vi "Queued Temperature Controller.vi"() -> ()   [LabVIEW 2013]
uses:
  Heater State.ctl
  <vilib>/Analysis/baseanly.llb/Mean (DBL).vi
  <vilib>/Analysis/NI_AALBase.lvlib
panel:
  out "Current Temperature":dbl
  out "History":dbl(graph)
  in  "Temperature Control":dbl(slide)=1994.949494949495 scale=0.0..2500.0
  out "Heating Boolean":bool
  out "Mean":dbl format="%0.2f"
  out "Current Mean":dbl
  out "Min value":dbl
  out "Max value":dbl
  in  "Stop Button":bool
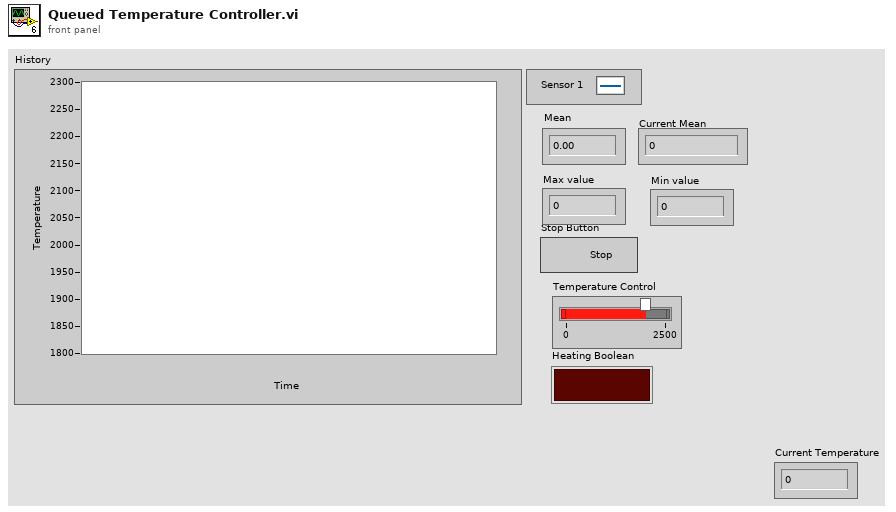
[diagram p1: front panel]
types:
  T1 = typedef "Heater State.ctl" = enum16{"Heater off", "Heating"}
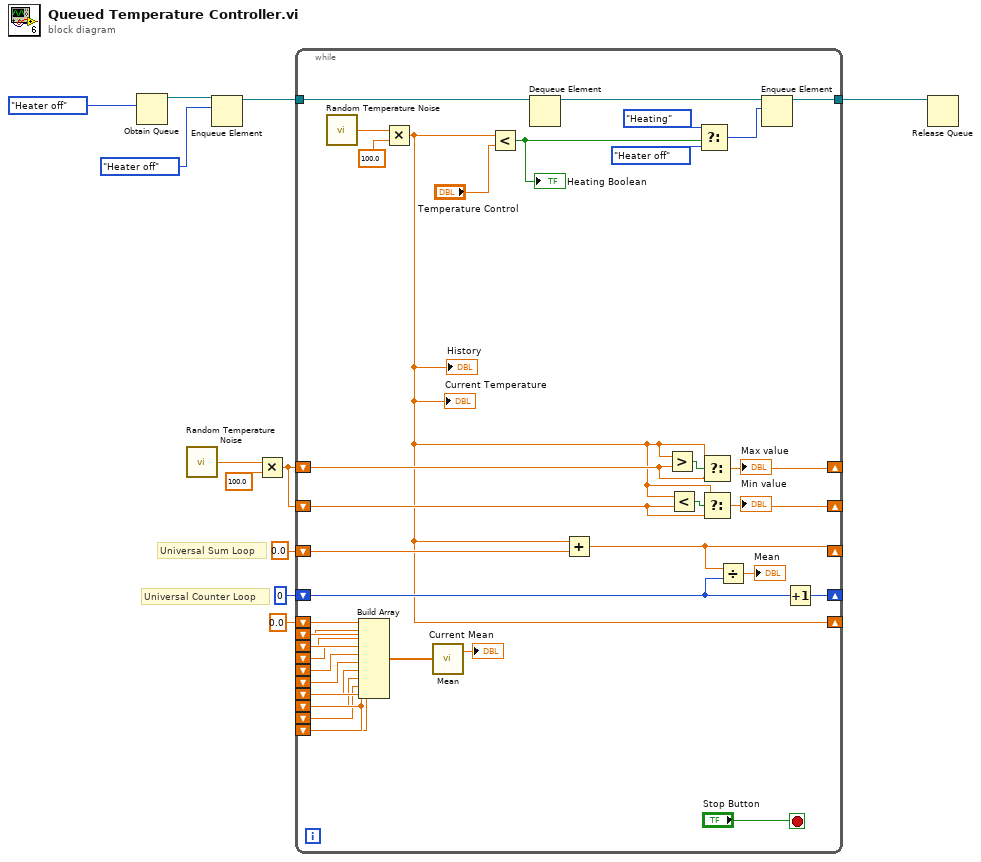
[diagram p0: block diagram]
diagram:
  w6 = 0.0
  # "Universal Sum Loop"
  # "Universal Counter Loop"
  n1 = Obtain Queue(element data type=Heater_State."Heater off" ("Heater State")) -> (queue out=w4:refnum<queue>)  [unwired: 4 in, 2 out]
  n2 = call "Random Temperature Noise.vi"() -> ("Temperature"=w10:dbl)  [unwired: 1 in]
  n3 = Enqueue Element(queue=w4, element=Heater_State."Heater off" ("Heater State")) -> (queue out=w2:refnum<queue>)  [unwired: 2 in, 2 out]
  n4 = Multiply(x=w10, y=100.0) -> (x*y=w8:dbl)
  n5 = while {
    shift-right: [w25] -> _
    shift-left: 0.0 -> [w24]
    shift-right: [w41] -> _
    shift-left: w8 -> [w39]
    shift-right: [w40] -> _
    shift-left: w8 -> [w38]
    shift-right: [w12] -> _
    shift-left: w6 -> [w35]
    shift-left: w6 -> [w34]
    shift-left: w6 -> [w26]
    shift-left: w6 -> [w33]
    shift-left: w6 -> [w28]
    shift-left: w6 -> [w29]
    shift-right: [w36] -> _
    shift-left: 0 -> [w22]
    shift-left: w6 -> [w27]
    shift-left: w6 -> [w32]
    shift-left: w6 -> [w30]
    shift-left: w6 -> [w31]
    tunnel: w2 -> [w19]
    tunnel: [w14] -> w1
    stop <- "Stop Button" stop-if-true
    n6 = call "Random Temperature Noise.vi"() -> ("Temperature"=w44:dbl)  [unwired: 1 in]
    n7 = Build Array(w35, w34, w33, w32, w31, w30, w29, w28, w27, w26) -> (w20:dbl[])
    n8 = Multiply(x=w44, y=100.0) -> (x*y=w12:dbl)
    "History" <- w12
    "Current Temperature" <- w12
    n9 = call-poly <vilib>:"Mean.vi"("X"=w20) -> ("mean"=→"Current Mean":dbl)  [unwired: 1 out]
    n10 = Less?(x=w12, y="Temperature Control") -> (x < y?=w16:bool)
    "Heating Boolean" <- w16
    n11 = Dequeue Element(queue=w19) -> (queue out=w18:refnum<queue>)  [unwired: 2 in, 3 out]
    n12 = Add(x=w12, y=w24) -> (x+y=w25:dbl)
    n13 = Greater?(x=w12, y=w39) -> (0:w43:bool)
    n14 = Less?(x=w12, y=w38) -> (x < y?=w42:bool)
    n15 = Select(t=Heater_State."Heating" ("Heater State"), s=w16, f=Heater_State."Heater off" ("Heater State")) -> (s? t:f=w15:T1)
    n16 = Select(t=w12, s=w43, f=w39) -> (s? t:f=w41:dbl)
    "Max value" <- w41
    n17 = Select(t=w12, s=w42, f=w38) -> (s? t:f=w40:dbl)
    "Min value" <- w40
    n18 = Divide(x=w25, y=w22) -> (x/y=→"Mean":dbl)
    n19 = Enqueue Element(queue=w18, element=w15) -> (queue out=w14:refnum<queue>)  [unwired: 2 in, 2 out]
    n20 = Increment(x=w22) -> (x+1=w36:i32)
  }
  n21 = Release Queue(queue=w1) -> ()  [unwired: 2 in, 3 out]
